vi "Configure Modulation (Custom).vi"(0 "VISA resource name":refnum<visa-resource-name>, 1 "Enable Custom Modulation (T:Enable)":bool=TRUE, 2 "MSK Phase Deviation (90 deg)":dbl=90.0, 3 "FSK Frequency Deviation (400 Hz)":dbl=400.0, 5 "Standard (0: None)":u16(ring) items=["None", "APCO 25 w/C4FM", "APCO 25 w/CQPSK", "Bluetooth", "CDPD"], 7 "Modulation Type (6: pi/4 DQPSK)":u16(ring)=6 items=["BPSK", "QPSK", "IS-95 QPSK", "Gray Coded QPSK", "OQPSK", "IS-95 OQPSK", "pi/4 DQPSK", "8PSK", "16PSK", "D8PSK", "MSK", "2-Lvl FSK", "4-Lvl FSK", "8-Lvl FSK", "16-Lvl FSK", "C4FM", "4QAM", "16QAM", "32QAM", "64QAM", "128QAM", "256QAM", "User I/Q", "User FSK", "ASK", "UQPSK", "EDGE", "1024QAM", "VSA 16QAM", "VSA 32QAM", "VSA 64QAM", "VSA 128QAM", "VSA 256QAM", "VSA 512QAM", "VSA 1024QAM"], 9 "File Name (\"\")":string, 11 "error in (no error)":errorcluster, 12 "Symbol Rate (24.3 kbps)":dbl=24300.0, 13 "I/Q Scaling (70 percent)":dbl=70.0, 14 "Phase Polarity (0: Normal)":u16(ring) items=["Normal", "Inverted"]) -> (4 "VISA resource name out":refnum<visa-resource-name>, 15 "error out":errorcluster)   [LabVIEW 2012, in "Agilent PSG MXG Series.lvlib"]
doc: "Configures the state, type, standard, phase polarity, I/Q scaling value and symbol rate for the custom modulation.\n\n<B>Notes:</B>\n(1) This VI is valid only in E8267C, E8267D, N5172B, N5182B.\n\n(2) For E8267C, this VI is valid only when the instrument installs <B>Option 002</B> (Internal baseband generator) or <B>Option 602</B> (Digital bus baseband generator).\n\n(3) For E8267D, this VI is valid only when the instrument installs <B>Option 601</B> or <B>Option 602</B> (Internal baseband generator).\n\n(4) For N5172B and N5182B, this VI is valid only when the instrument installs <B>Option 431</B>."
uses:
  <instrlib>/Agilent PSG MXG Series/Agilent PSG MXG Series.lvlib
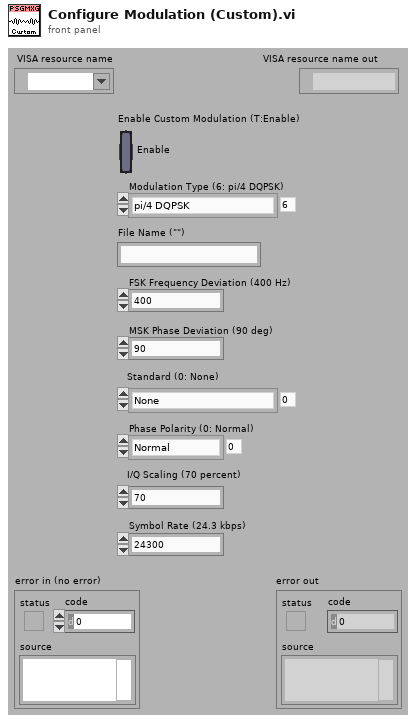
[diagram p1: front panel]
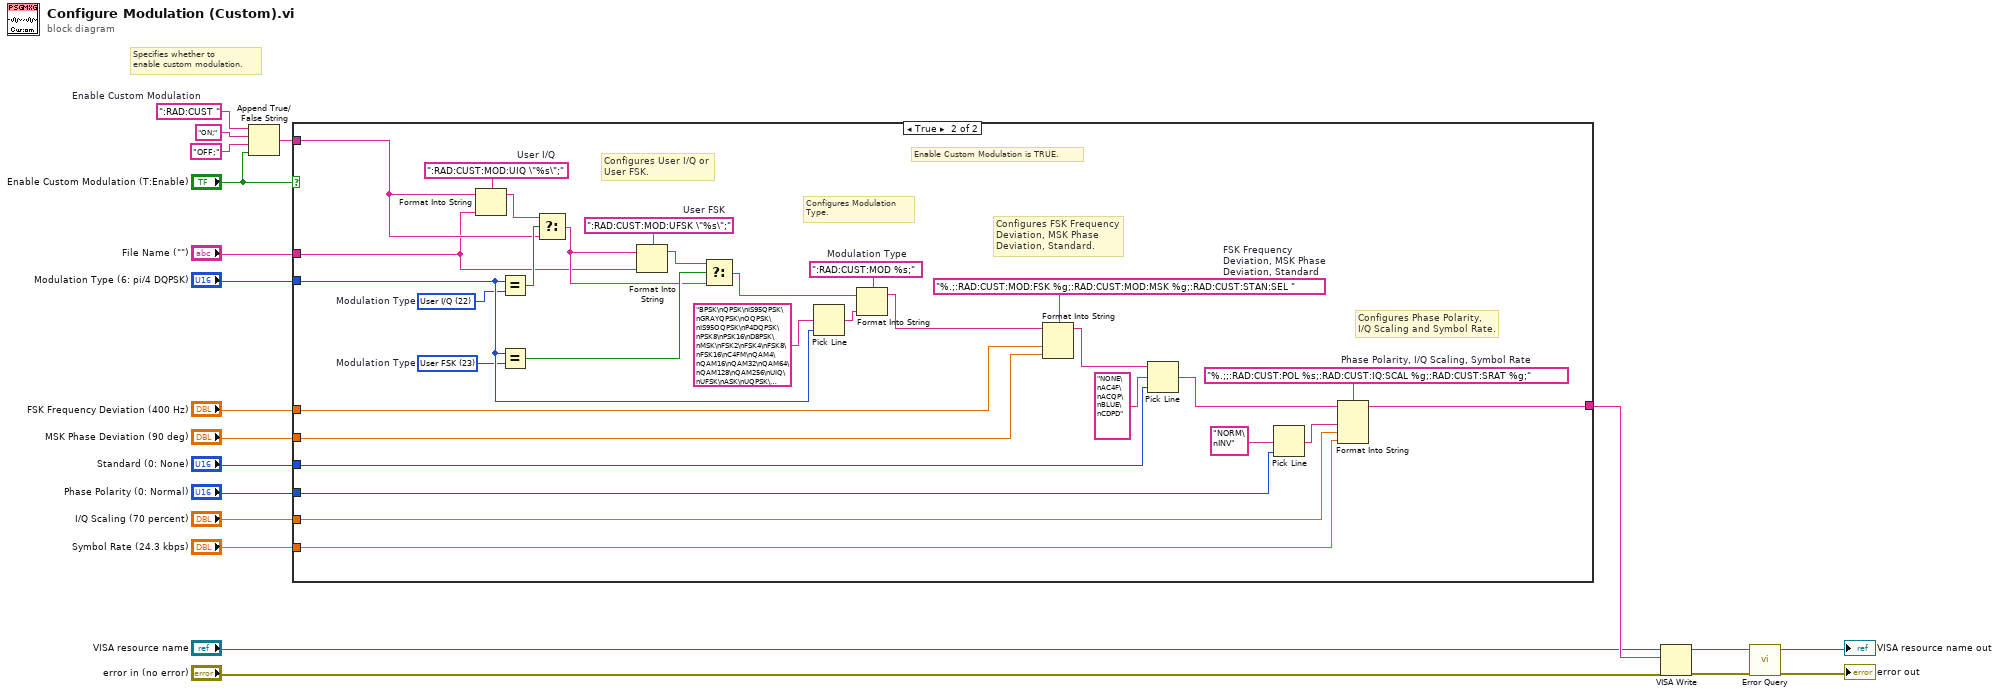
[diagram p0: block diagram]
diagram:
  w20 = ":RAD:CUST "  # Enable Custom Modulation
  # "Specifies whether to\nenable custom modulation."
  n1 = Append True/False String(1:"Enable Custom Modulation (T:Enable)", 2:"OFF;" ("false string"), 3:"ON;" ("true string"), 4:w20) -> (0:w16:string)
  n2 = case shown="True" "Enable Custom Modulation (T:Enable)" {
    tunnel: w16 -> [w21 w32]
    tunnel: "Modulation Type (6: pi/4 DQPSK)" -> [_ w25]
    tunnel: "File Name (\"\")" -> [_ w30]
    tunnel: "FSK Frequency Deviation (400 Hz)" -> [_ w45]
    tunnel: "MSK Phase Deviation (90 deg)" -> [_ w44]
    tunnel: "Standard (0: None)" -> [_ w41]
    tunnel: "Phase Polarity (0: Normal)" -> [_ w36]
    tunnel: "I/Q Scaling (70 percent)" -> [_ w35]
    tunnel: "Symbol Rate (24.3 kbps)" -> [_ w34]
    tunnel: [w21 w33] -> w7
    frame False {
      # "Enable Custom Modulation\nis FALSE."
    }
    frame True {
      w22 = u16 23 items=["BPSK", "QPSK", "IS-95 QPSK", "Gray Coded QPSK", "OQPSK", "IS-95 OQPSK", "pi/4 DQPSK", "8PSK", "16PSK", "D8PSK", "MSK", "2-Lvl FSK", "4-Lvl FSK", "8-Lvl FSK", "16-Lvl FSK", "C4FM", "4QAM", "16QAM", "32QAM", "64QAM", "128QAM", "256QAM", "User I/Q", "User FSK", "ASK", "UQPSK", "EDGE", "1024QAM", "VSA 16QAM", "VSA 32QAM", "VSA 64QAM", "VSA 128QAM", "VSA 256QAM", "VSA 512QAM", "VSA 1024QAM"]  # Modulation Type
      w23 = u16 22 items=["BPSK", "QPSK", "IS-95 QPSK", "Gray Coded QPSK", "OQPSK", "IS-95 OQPSK", "pi/4 DQPSK", "8PSK", "16PSK", "D8PSK", "MSK", "2-Lvl FSK", "4-Lvl FSK", "8-Lvl FSK", "16-Lvl FSK", "C4FM", "4QAM", "16QAM", "32QAM", "64QAM", "128QAM", "256QAM", "User I/Q", "User FSK", "ASK", "UQPSK", "EDGE", "1024QAM", "VSA 16QAM", "VSA 32QAM", "VSA 64QAM", "VSA 128QAM", "VSA 256QAM", "VSA 512QAM", "VSA 1024QAM"]  # Modulation Type
      w27 = ":RAD:CUST:MOD %s;"  # Modulation Type
      w39 = "%.;;:RAD:CUST:POL %s;:RAD:CUST:IQ:SCAL %g;:RAD:CUST:SRAT %g;"  # Phase Polarity, I/Q Scaling, Symbol Rate
      w46 = "%.;:RAD:CUST:MOD:FSK %g;:RAD:CUST:MOD:MSK %g;:RAD:CUST:STAN:SEL "  # FSK Frequency Deviation, MSK Phase Deviation, Standard
      w49 = ":RAD:CUST:MOD:UFSK \"%s\";"  # User FSK
      w52 = ":RAD:CUST:MOD:UIQ \"%s\";"  # User I/Q
      # "Configures Phase Polarity,\nI/Q Scaling and Symbol Rate."
      # "Configures FSK Frequency\nDeviation, MSK Phase\nDeviation, Standard."
      # "Configures Modulation\nType."
      # "Configures User I/Q or\nUser FSK."
      # "Enable Custom Modulation is TRUE."
      n3 = Format Into String(format string=w52, initial string=w32, w30) -> (resulting string=w50:string)  [unwired: 1 in, 1 out]
      n4 = Equal?(x=w25, y=w23) -> (x = y?=w51:bool)
      n5 = Equal?(x=w25, y=w22) -> (x = y?=w48:bool)
      n6 = Select(t=w50, s=w51, f=w32) -> (s? t:f=w47:string)
      n7 = Format Into String(format string=w49, initial string=w47, w30) -> (resulting string=w31:string)  [unwired: 1 in, 1 out]
      n8 = Select(t=w31, s=w48, f=w47) -> (s? t:f=w28:string)
      n9 = Pick Line(multi-line string="BPSK\nQPSK\nIS95QPSK\nGRAYQPSK\nOQPSK\nIS95OQPSK\nP4DQPSK\nPSK8\nPSK16\nD8PSK\nMSK\nFSK2\nFSK4\nFSK8\nFSK16\nC4FM\nQAM4\nQAM16\nQAM32\nQAM64\nQAM128\nQAM256\nUIQ\nUFSK\nASK\nUQPSK\nEDGE\nQAM1024\nVSAQAM16\nVSAQAM32\nVSAQAM64\nVSAQAM128\nVSAQAM256\nVSAQAM512\nVSAQAM1024", line index=w25) -> (output string=w29:string)  [unwired: 1 out]
      n10 = Format Into String(format string=w27, initial string=w28, w29) -> (resulting string=w24:string)  [unwired: 1 in, 1 out]
      n11 = Format Into String(format string=w46, initial string=w24, w45, w44) -> (resulting string=w43:string)  [unwired: 1 in, 1 out]
      n12 = Pick Line(string ("")=w43, multi-line string="NONE\nAC4F\nACQP\nBLUE\nCDPD", line index=w41) -> (output string=w40:string)
      n13 = Pick Line(multi-line string="NORM\nINV", line index=w36) -> (output string=w38:string)  [unwired: 1 out]
      n14 = Format Into String(format string=w39, initial string=w40, w38, w35, w34) -> (resulting string=w33:string)  [unwired: 1 in, 1 out]
    }
  }
  n15 = VISA Write(VISA resource name="VISA resource name", write buffer=w7, error in (no error)="error in (no error)") -> (VISA resource name out=w6:refnum<visa-resource-name>, error out=w5:errorcluster)  [unwired: 1 out]
  n16 = call <instrlib>:"Error Query.vi"("error in (no error)"=w5, "VISA resource name"=w6) -> ("error out"=→"error out":errorcluster, "VISA resource name out"=→"VISA resource name out":refnum<visa-resource-name>)  [unwired: 8 out]
